vi "Begin_TipperV2.vi"() -> ()   [LabVIEW 2011]
uses:
  <vilib>/Rock Robotics/WPI/CAN/Jaguar/SubVIs/WPI_CANJaguar_BrakeCoastMode.ctl
  <vilib>/Rock Robotics/SystemInterfaces/AI/FPGA_AIChannel.ctl
  <vilib>/Rock Robotics/SystemInterfaces/Typedef/FPGA_TypedefAnalogModule.ctl
  <vilib>/Rock Robotics/WPI/MotorControl/WPI_MotorControlOpenCANJaguar.vi
panel:
  out "error out":T1
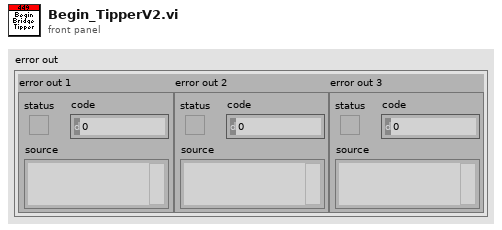
[diagram p1: front panel]
types:
  T1 = cluster{"error out 1":errorcluster, "error out 2":errorcluster, "error out 3":errorcluster}
  T2 = typedef "FPGA_AIChannel.ctl" = enum8{"AI 1", "AI 2", "AI 3", "AI 4", "AI 5", "AI 6", "AI 7", "AI 8", "Invalid"}
  T3 = typedef "FPGA_TypedefAnalogModule.ctl" = enum16{"Analog Module 1", "Analog Module 2"}
  T4 = typedef "WPI_CANJaguar_BrakeCoastMode.ctl" = enum8{"Jumper", "Brake", "Coast"}
  T5 = typedef "WPI_MotorControlDeviceRef.ctl" = cluster{"DeviceStatus":errorcluster, "Type":enum16{"PWM", "CAN"}, "PWM":cluster{"Digital Module":T6, "PWM Channel":T7, "DeadBand":T8}, "CAN":cluster{"Device Number":u8, "Control Mode":T9, "Semaphore":T10, "Max Vout":dbl}, "Invert":bool, "TransformRef":T11, "InvTransformRef":T11}
  T6 = typedef "FPGA_TypedefDigitalModule.ctl" = enum16{"Digital Module 1", "Digital Module 2"}
  T7 = typedef "FPGA_DIOPWMChannel.ctl" = enum8{"PWM 1", "PWM 2", "PWM 3", "PWM 4", "PWM 5", "PWM 6", "PWM 7", "PWM 8", "PWM 9", "PWM 10", "Invalid"}
  T8 = typedef "WPI_PWMDeadband.ctl" = cluster{"Name":string, "maxPositivePwm":i32, "minPositivePwm":i32, "centerPwm":i32, "maxNegativePwm":i32, "minNegativePwm":i32, "angularRange":u16}
  T9 = typedef "WPI_CANJaguar_ControlMode.ctl" = enum8{"Percent VBus", "Current", "Speed", "Position", "Voltage"}
  T10 = typedef "Semaphore RefNum" = refnum<k1>
  T11 = typedef "WPI_PWMTransform_ConPane.ctl" = refnum<vi>
  T12 = typedef "WPI_AnalogChannelDevRef.ctl" = cluster{"DevStatus":errorcluster, "Analog Module":T3, "Analog Channel":T2}
  T13 = cluster{"error out":errorcluster, "error out":errorcluster, "error out":errorcluster}
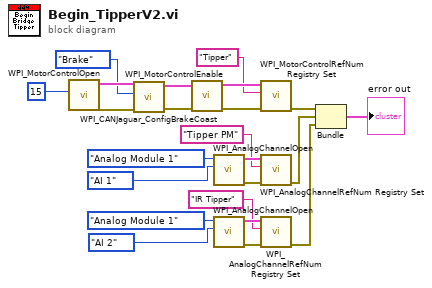
[diagram p0: block diagram]
diagram:
  n1 = call-poly <vilib>:"WPI_MotorControlOpen.vi"("Device Number"=u8 15) -> ("error out"=w17:errorcluster, "MotorControlDeviceRef"=w16:T5)  [unwired: 9 in]
  n2 = call <vilib>:"WPI_CANJaguar_ConfigBrakeCoast.vi"("error in (no error)"=w17, "Brake / Coast Mode"=WPI_CANJaguar_BrakeCoastMode."Brake", "CAN Jaguar Ref"=w16) -> ("error out"=w18:errorcluster, "CAN Jaguar Ref Out"=w19:T5)  [unwired: 7 in]
  n3 = call <vilib>:"WPI_MotorControlEnable.vi"("error in (no error)"=w18, "CAN Jaguar Ref"=w19) -> ("error out"=w22:errorcluster, "CAN Jaguar Ref Out"=w21:T5)  [unwired: 8 in]
  n4 = call <vilib>:"WPI_AnalogChannelOpen.vi"("Analog Channel"=FPGA_AIChannel."AI 1", "Analog Module (Module 1)"=FPGA_TypedefAnalogModule."Analog Module 1") -> ("error out"=w12:errorcluster, "AIDeviceRef"=w11:T12)  [unwired: 8 in]
  n5 = call <vilib>:"WPI_AnalogChannelOpen.vi"("Analog Channel"=FPGA_AIChannel."AI 2", "Analog Module (Module 1)"=FPGA_TypedefAnalogModule."Analog Module 1") -> ("error out"=w3:errorcluster, "AIDeviceRef"=w4:T12)  [unwired: 8 in]
  n6 = call <vilib>:"WPI_MotorControlRefNum Registry Set.vi"("error in (no error)"=w22, "refnum name"="Tipper", "MotorControlDevRef"=w21) -> ("error out"=w9:errorcluster)  [unwired: 7 in, 1 out]
  n7 = call <vilib>:"WPI_AnalogChannelRefNum Registry Set.vi"("error in (no error)"=w12, "refnum name"="Tipper PM", "AIDeviceRef"=w11) -> ("error out"=w8:errorcluster)  [unwired: 7 in, 1 out]
  n8 = call <vilib>:"WPI_AnalogChannelRefNum Registry Set.vi"("error in (no error)"=w3, "refnum name"="IR Tipper", "AIDeviceRef"=w4) -> ("error out"=w1:errorcluster)  [unwired: 7 in, 1 out]
  n9 = Bundle("error out"=w9, "error out"=w8, "error out"=w1) -> (→"error out":T13)  [unwired: 1 in]
